vi "Periodic Tasks.vi"(8 "error in":errorcluster) -> ()   [LabVIEW 2016]
doc: "This VI runs in parallel to other tasks. It can contain as many user-defined periodic loops as you need. These can carry out PID or other sorts of timed response."
uses:
  <vilib>/Rock Robotics/WPI/Utilities/WPI_GetSetVariantRefNum.vi
  Robot Global Data.vi
  <vilib>/Rock Robotics/Network Tables/NT Write Numeric Array.vi
  <vilib>/Rock Robotics/Network Tables/NT Write Number.vi
  <vilib>/Rock Robotics/WPI/Solenoid/WPI_SolenoidValue.ctl
  <vilib>/Rock Robotics/WPI/Solenoid/WPI_SolenoidSetEnum.vi
panel:
  in  "z axis offset":dbl=0.10000000000000006
  out "Waveform Chart":dbl[][](graph)=[[-62.41187234999887, 0.0]]
  in  "Right False":dbl=0.3
  in  "Left False":dbl=0.7
  in  "Right True":dbl=0.7
  in  "Left-True":dbl=0.3 format="%#_13g"
  out "SensorPosRotations":dbl=1921.607142857143
  out "Motor output Plot 2":cluster{"Applied Throttle":dbl}(graph)
  out "Target RPM":dbl=5349.336450505878
  out "SensorRPM Velocity RPM 2":dbl
  in  "Ramp Rate 2":dbl
  in  "I Zone 2":dbl
  in  "D 2":dbl=-0.008
  in  "I 2":dbl=-0.027
  in  "P 2":dbl=20.0
  out "Applied Output 2":dbl
  out "Speed Closed Loop Plots":T1(graph)={"Sensor Velocity"=0.0, "Encoder Velocity"=0.0, "Encoder Position"=-53805.0}
  out "SensorPos (rotations)":dbl=-0.15048543689320387
  out "Motor output Plot":cluster{"Applied Throttle":dbl}(graph)
  out "Target Position (rotations)":dbl=-0.15274800672560607
  out "SensorRPM Velocity RPM":dbl
  in  "Ramp Rate":dbl=2.0
  in  "I Zone":dbl
  in  "F - Generally is zero for position-servo":dbl
  in  "D":dbl=0.45
  in  "I":dbl=0.0001
  in  "P":dbl=1.9
  out "Applied Output":dbl
  out "Position Closed Loop Plots":cluster{dbl, "Sensor Velocity":dbl}(graph)={1.352755905511811, "Sensor Velocity"=1.3564954682779455}
  out "rightDistance":dbl=27.365850000000002
  out "leftDistance":dbl=-30.4065
  # "Launcher Control"
  # "Turret Controls"
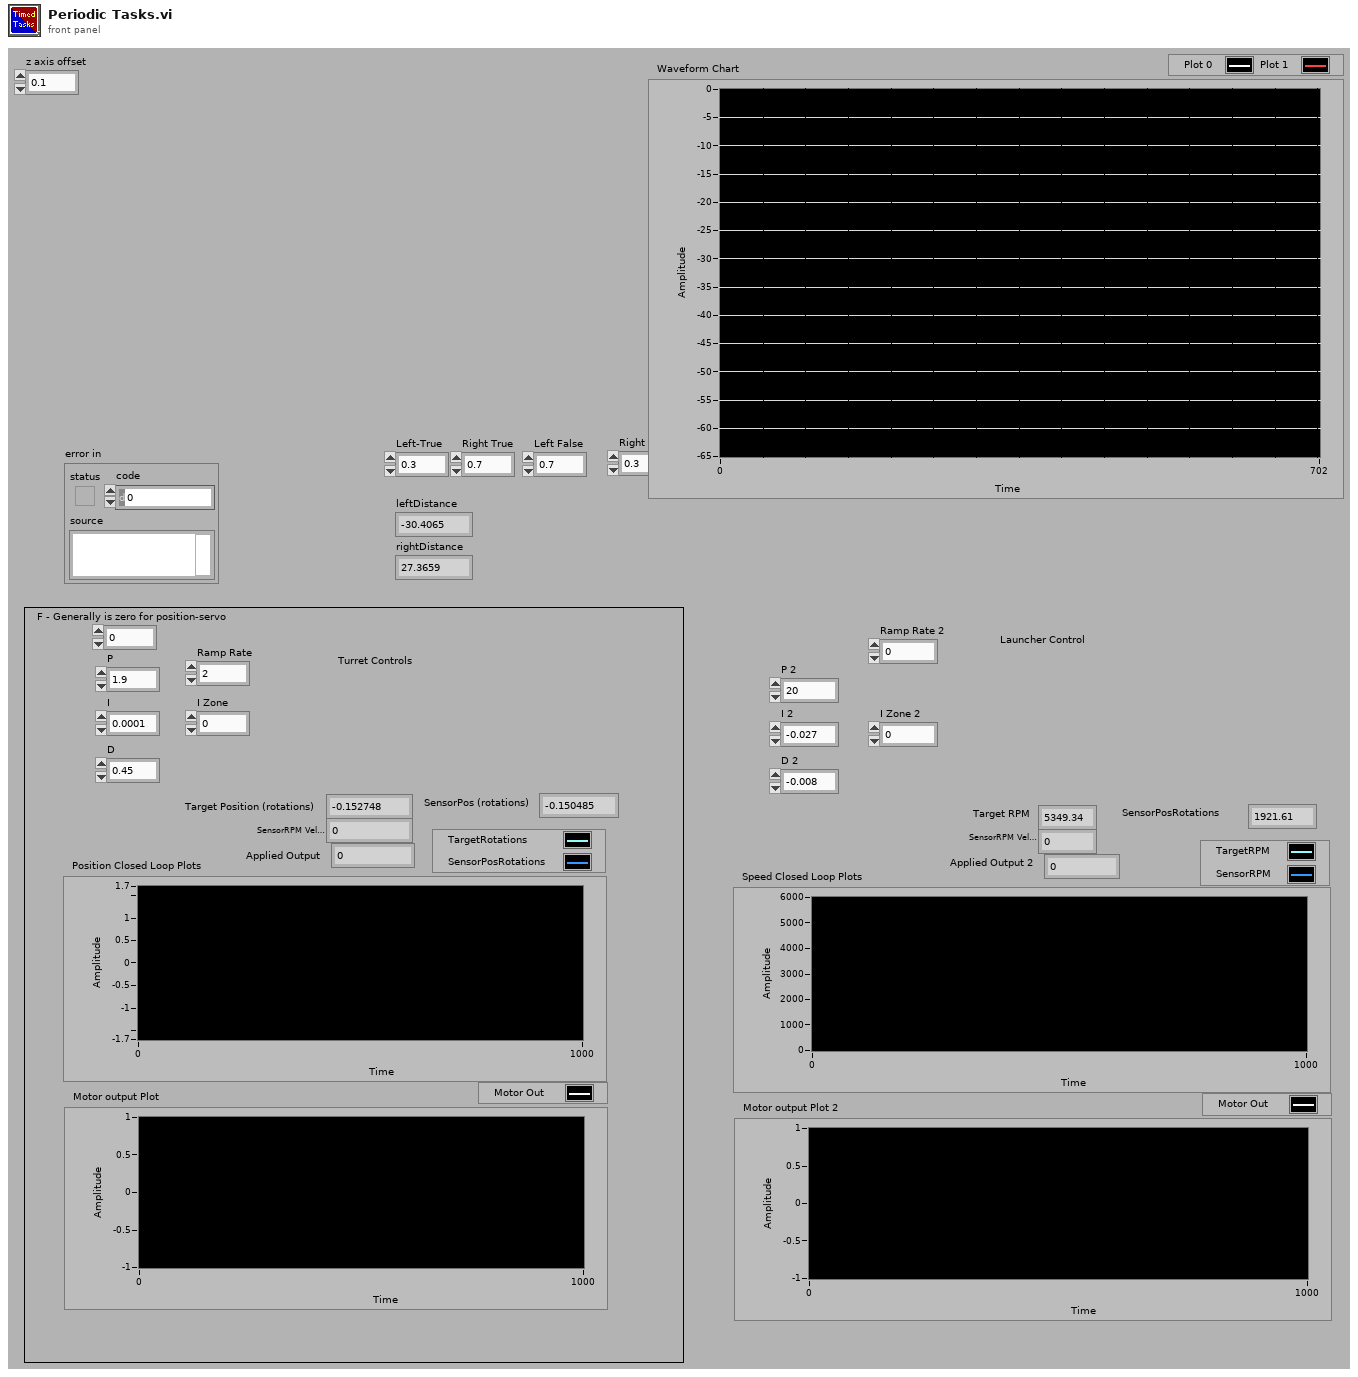
[diagram p1: front panel]
types:
  T1 = cluster{"Sensor Velocity":dbl, "Encoder Velocity":dbl, "Encoder Position":dbl}
  T2 = typedef "WPI_ServoDeviceRef.ctl" = cluster{"DeviceStatus":errorcluster, "PWM Channel":T3, "DeadBand":T4}
  T3 = typedef "FPGA_DIOPWMChannel.ctl" = enum8{"PWM 0", "PWM 1", "PWM 2", "PWM 3", "PWM 4", "PWM 5", "PWM 6", "PWM 7", "PWM 8", "PWM 9", "PWM MXP 0", "PWM MXP 1", "PWM MXP 2", "PWM MXP 3", "PWM MXP 4", "PWM MXP 5", "PWM MXP 6", "PWM MXP 7", "PWM MXP 8", "PWM MXP 9", "Invalid"}
  T4 = typedef "WPI_PWMDeadband.ctl" = cluster{"Name":string, "maxPositivePwm":i32, "minPositivePwm":i32, "centerPwm":i32, "maxNegativePwm":i32, "minNegativePwm":i32, "angularRange":u16}
  T5 = typedef "WPI_SolenoidValue.ctl" = enum16{"Off", "On", "Forward", "Reverse"}
  T6 = typedef "WPI_SolenoidDevRef.ctl" = cluster{"DevStatus":errorcluster, "Pneumatics Control Module":u8, "Forward Solenoid Channel":T7, "Reverse Solenoid Channel":T7}
  T7 = typedef "WPI_SolenoidChannel.ctl" = enum8{"Solenoid 0", "Solenoid 1", "Solenoid 2", "Solenoid 3", "Solenoid 4", "Solenoid 5", "Solenoid 6", "Solenoid 7", "Invalid"}
  T8 = typedef "WPI_MotorControlDeviceRef.ctl" = cluster{"DeviceStatus":errorcluster, "Type":T9, "PWM":cluster{"PWM Channel":T3, "DeadBand":T4}, "CAN":cluster{"Device Number":u8, "SetOutput VI Ref":variant, "GetOutput VI Ref":variant, "Enable VI Ref":variant, "Disable VI Ref":variant, "Data":variant}, "Invert":bool}
  T9 = typedef "WPI_MotorControlType.ctl" = enum16{"PWM", "CAN"}
  T10 = typedef "WPI_RobotDriveDevRef.ctl" = cluster{"DevStatus":errorcluster, "Motors[]":T8[], "Square Inputs":bool, "Max Output":dbl}
  T11 = typedef "WPI_GyroDevRef.ctl" = cluster{"DevStatus":errorcluster, "Analog Channel":T12, "Offset":dbl, "Gain (VoltsPerDegree/Second)":dbl, "Gyro Type":enum16{"Analog", "XRS450"}, "Handle":i32, "SPI Bus":T13, "Device Found":bool, "Sample Rate":dbl, "Calibrate On Open":bool}
  T12 = typedef "FPGA_AIChannel.ctl" = enum8{"AI 0", "AI 1", "AI 2", "AI 3", "AI MXP 0", "AI MXP 1", "AI MXP 2", "AI MXP 3", "Invalid"}
  T13 = typedef "spi_bus.ctl" = enum16{"SPI On-Board, CS0", "SPI On-Board, CS1", "SPI On-Board, CS2", "SPI On-Board, CS3", "SPI MXP", "Invalid"}
  T14 = typedef "WPI_EncoderDevRef.ctl" = cluster{"DevStatus":errorcluster, "EncoderIndex":T15, "CounterIndex":T16, "DistancePerCount":dbl, "Decoding Type":T17}
  T15 = typedef "FPGA_EncoderIdx.ctl" = enum8{"Enc 0", "Enc 1", "Enc 2", "Enc 3", "Enc 4", "Enc 5", "Enc 6", "Enc 7", "Invalid"}
  T16 = typedef "FPGA_CounterCtrSystemIndex.ctl" = enum8{"Ctr 0", "Ctr 1", "Ctr 2", "Ctr 3", "Ctr 4", "Ctr 5", "Ctr 6", "Ctr 7", "Invalid"}
  T17 = typedef "WPI_EncoderType.ctl" = enum16{"1x", "2x", "4x"}
  T18 = typedef "WPI_CANTalonSRX_GlobalStatus.ctl" = cluster{"Applied Throttle":dbl, "Module Enabled":bool, "CAN Error":errorcluster, "Closed Loop Error":dbl, "Forward Limit Switch Closed":bool, "Reverse Limit Switch Closed":bool, "Sensor Position":dbl, "Sensor Velocity":dbl, "Current":dbl, "Sticky Fault - Over Temp":bool, "Sticky Fault - Under Voltage":bool, "Sticky Fault - Forward Limit":bool, "Sticky Fault - Reverse Limit":bool, "Sticky Fault - Forward Soft Limit":bool, "Sticky Fault - Reverse Soft Limit":bool, "Brake is Enabled":bool, "Encoder Position":dbl, "Encoder Velocity":dbl, "Encoder Index Count":dbl, "Encoder A Pin State":bool, "Encoder B Pin State":bool, "Encoder Index Pin State":bool, "Analog In":dbl, "Analog In Velocity":dbl, "Temperature (C)":dbl, "Battery Voltage":dbl, "Control 5 Is Supported":bool, "Current Profile Slot Select":dbl, "Pos Div 8":bool, "Vel Div 4":bool, "Pulse Width Position":i32, "Pulse Width Velocity":i32, "Pulse Width Rise To Rise (us)":i32, "Pulse Width Rise To Fall (us)":i32, "Mot Prof Active Is Under Run":bool, "Mot Prof Active Has Under Run":bool, "Mot Prof Active Is Last":bool, "Mot Prof Active Velocity Only":bool, "Mot Prof Active Is Valid":bool, "Mot Prof Buffer Is Full":bool, "Mot Prof Active Profile Slot Select":i32, "Mot Prof NextID":i32, "Mot Prof Count":i32, "Mot Prof Active Velocity":dbl, "Mot Prof Active Position":dbl, "Mot Prof Output Enable":i32, "UsageFrame":u32, "Motion Magic Active Trajectory":cluster{"Velocity":dbl, "Position":dbl}}
  T19 = typedef "WPI_SwitchDevRef.ctl" = cluster{"DevStatus":errorcluster, "DIO Channel":T20, "CntIndex":T16, "Normally Closed":bool}
  T20 = typedef "FPGA_DIOChannel.ctl" = enum8{"DIO 0", "DIO 1", "DIO 2", "DIO 3", "DIO 4", "DIO 5", "DIO 6", "DIO 7", "DIO 8", "DIO 9", "DIO MXP 0", "DIO MXP 1", "DIO MXP 2", "DIO MXP 3", "DIO MXP 4", "DIO MXP 5", "DIO MXP 6", "DIO MXP 7", "DIO MXP 8", "DIO MXP 9", "DIO MXP 10", "DIO MXP 11", "DIO MXP 12", "DIO MXP 13", "DIO MXP 14", "DIO MXP 15", "SPI Port CS1", "SPI Port CS2", "SPI Port CS3", "SPI Port MISO", "SPI Port MOSI", "Invalid"}
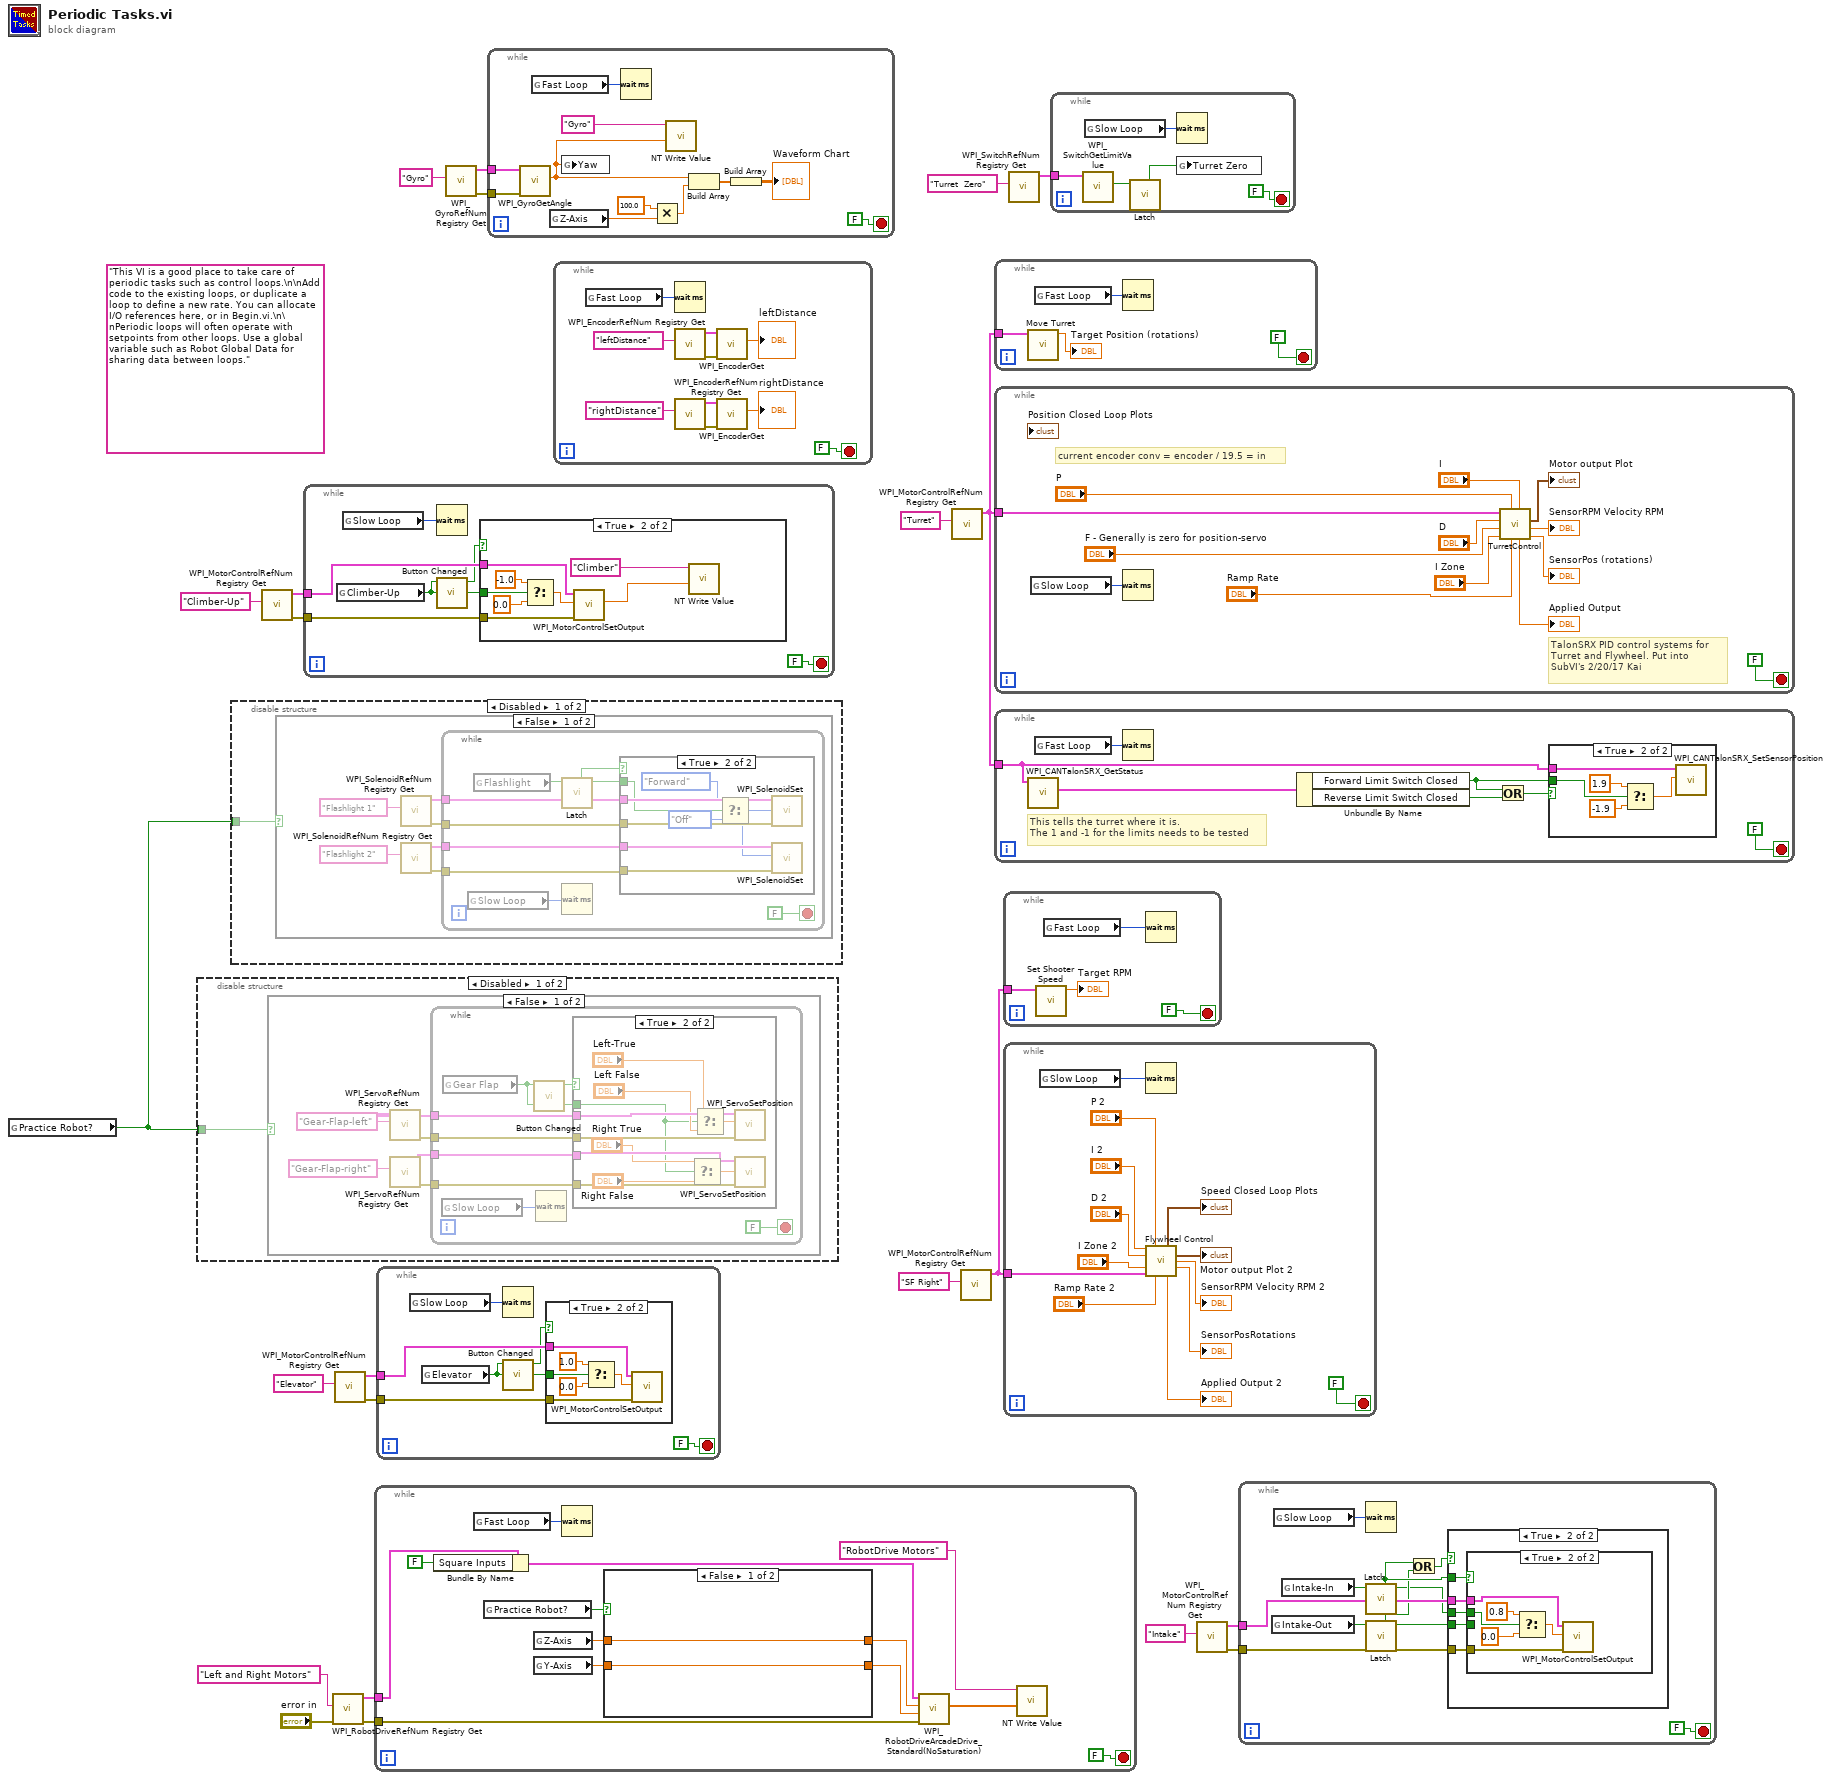
[diagram p0: block diagram]
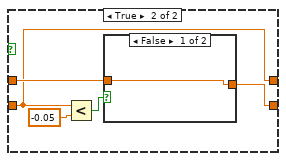
[diagram p10: hidden frame]
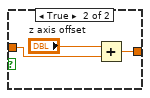
[diagram p11: hidden frame]
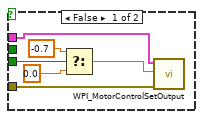
[diagram p14: hidden frame]
diagram:
  (unwired) "This VI is a good place to take care of periodic tasks such as control loops.\n\nAdd code to the existing loops, or duplicate a loop to define a new rate. You can allocate I/O references here, or in Begin.vi.\n\nPeriodic loops will often operate with setpoints from other loops. Use a global variable such as Robot Global Data for sharing data between loops."
  n1 = global read "Robot Global Data.vi" "Practice Robot?"() -> (w13:bool)
  n2 = disable-structure shown="Disabled" {
    disable-tunnel: w13 -> [w24 _]
    frame Disabled {
      n3 = case shown="False" w24 {
        frame False {
          n4 = call <vilib>:"WPI_ServoRefNum Registry Get.vi"("refnum name"="Gear-Flap-left") -> ("error out"=w27:errorcluster, "ServoDeviceRef"=w28:T2)  [unwired: 9 in]
          n5 = call <vilib>:"WPI_ServoRefNum Registry Get.vi"("refnum name"="Gear-Flap-right") -> ("error out"=w25:errorcluster, "ServoDeviceRef"=w26:T2)  [unwired: 9 in]
          n6 = while {
            tunnel: w28 -> [w38]
            tunnel: w27 -> [w37]
            tunnel: w26 -> [w36]
            tunnel: w25 -> [w35]
            stop <- FALSE stop-if-true
            n7 = global read "Robot Global Data.vi" "Slow Loop"() -> (w34:u32)
            n8 = global read "Robot Global Data.vi" "Gear Flap"() -> (w32:bool)
            n9 = call "Button Changed.vi"("In"=w32) -> ("button changed"=w33:bool)  [unwired: 10 in]
            n10 = Wait (ms)(milliseconds to wait=w34) -> ()  [unwired: 1 out]
            n11 = case shown="True" w33 {
              tunnel: w38 -> [_ w49]
              tunnel: w37 -> [_ w48]
              tunnel: w36 -> [_ w47]
              tunnel: w35 -> [_ w46]
              tunnel: w32 -> [_ w40]
              frame False {
              }
              frame True {
                n12 = Select(t="Right True", s=w40, f="Right False") -> (s? t:f=w45:dbl)
                n13 = Select(t="Left-True", s=w40, f="Left False") -> (s? t:f=w42:dbl)
                n14 = call <vilib>:"WPI_ServoSetPosition.vi"("error in (no error)"=w48, "Position"=w42, "ServoDeviceRef"=w49) -> ()  [unwired: 7 in, 2 out]
                n15 = call <vilib>:"WPI_ServoSetPosition.vi"("error in (no error)"=w46, "Position"=w45, "ServoDeviceRef"=w47) -> ()  [unwired: 7 in, 2 out]
              }
            }
          }
        }
        frame True {
        }
      }
    }
    frame Enabled {
    }
  }
  n16 = disable-structure shown="Disabled" {
    disable-tunnel: w13 -> [w50 _]
    frame Disabled {
      n17 = case shown="False" w50 {
        frame False {
          n18 = call <vilib>:"WPI_SolenoidRefNum Registry Get.vi"("refnum name"="Flashlight 1") -> ("error out"=w53:errorcluster, "SolenoidDevRef"=w54:T6)  [unwired: 9 in]
          n19 = call <vilib>:"WPI_SolenoidRefNum Registry Get.vi"("refnum name"="Flashlight 2") -> ("error out"=w51:errorcluster, "SolenoidDevRef"=w52:T6)  [unwired: 9 in]
          n20 = while {
            tunnel: w54 -> [w62]
            tunnel: w53 -> [w61]
            tunnel: w52 -> [w60]
            tunnel: w51 -> [w59]
            stop <- FALSE stop-if-true
            n21 = global read "Robot Global Data.vi" "Slow Loop"() -> (w58:u32)
            n22 = global read "Robot Global Data.vi" "Flashlight"() -> (w63:bool)
            n23 = call "Latch.vi"("In"=w63) -> ("Out"=w65:bool, "button pressed"=w64:bool)  [unwired: 9 in]
            n24 = Wait (ms)(milliseconds to wait=w58) -> ()  [unwired: 1 out]
            n25 = case shown="True" w64 {
              tunnel: w62 -> [_ w73]
              tunnel: w61 -> [_ w72]
              tunnel: w60 -> [_ w71]
              tunnel: w59 -> [_ w70]
              tunnel: w65 -> [_ w67]
              frame False {
              }
              frame True {
                n26 = Select(t=WPI_SolenoidValue."Forward" ("Value"), s=w67, f=WPI_SolenoidValue."Off" ("Value")) -> (s? t:f=w66:T5)
                n27 = call-poly <vilib>:"WPI_SolenoidSet.vi"("error in (no error)"=w72, "Value"=w66, "SolenoidDevRef"=w73) -> ()  [unwired: 7 in, 2 out]
                n28 = call-poly <vilib>:"WPI_SolenoidSet.vi"("error in (no error)"=w70, "Value"=w66, "SolenoidDevRef"=w71) -> ()  [unwired: 7 in, 2 out]
              }
            }
          }
        }
        frame True {
        }
      }
    }
    frame Enabled {
    }
  }
  n29 = call <vilib>:"WPI_MotorControlRefNum Registry Get.vi"("refnum name"="Climber-Up") -> ("error out"=w14:errorcluster, "MotorControlDevRef"=w15:T8)  [unwired: 9 in]
  n30 = while {
    tunnel: w15 -> [w79]
    tunnel: w14 -> [w78]
    stop <- FALSE stop-if-true
    n31 = global read "Robot Global Data.vi" "Climber-Up"() -> (w74:bool)
    n32 = global read "Robot Global Data.vi" "Slow Loop"() -> (w77:u32)
    n33 = Wait (ms)(milliseconds to wait=w77) -> ()  [unwired: 1 out]
    n34 = call "Button Changed.vi"("In"=w74) -> ("button changed"=w76:bool)  [unwired: 10 in]
    n35 = case shown="True" w76 {
      tunnel: w79 -> [_ w87]
      tunnel: w78 -> [_ w86]
      tunnel: w74 -> [_ w83]
      frame False {
      }
      frame True {
        n36 = Select(t=-1.0 ("Motor Output"), s=w83, f=0.0 ("Motor Output")) -> (s? t:f=w81:dbl)
        n37 = call <vilib>:"WPI_MotorControlSetOutput.vi"("error in (no error)"=w86, "Output"=w81, "MotorControlDevRef"=w87) -> ("Motor Output"=w80:dbl)  [unwired: 6 in, 2 out]
        n38 = call-poly <vilib>:"NT Write Value.vi"("Numeric"=w80, "Name"="Climber") -> ()  [unwired: 9 in, 1 out]
      }
    }
  }
  n39 = call <vilib>:"WPI_RobotDriveRefNum Registry Get.vi"("error in (no error)"="error in", "refnum name"="Left and Right Motors") -> ("error out"=w9:errorcluster, "RobotDriveDevRef"=w10:T10)  [unwired: 8 out]
  n40 = call <vilib>:"WPI_MotorControlRefNum Registry Get.vi"("refnum name"="Elevator") -> ("error out"=w12:errorcluster, "MotorControlDevRef"=w11:T8)  [unwired: 9 in]
  n41 = while {
    tunnel: w10 -> [w98]
    tunnel: w9 -> [w97]
    stop <- FALSE stop-if-true
    n42 = Bundle By Name(cluster=w98, "Square Inputs"=FALSE) -> (w94:T10)
    n43 = global read "Robot Global Data.vi" "Fast Loop"() -> (w95:u32)
    n44 = global read "Robot Global Data.vi" "Practice Robot?"() -> (w88:bool)
    n45 = global read "Robot Global Data.vi" "Z-Axis"() -> (w92:dbl)
    n46 = global read "Robot Global Data.vi" "Y-Axis"() -> (w90:dbl)
    n47 = Wait (ms)(milliseconds to wait=w95) -> ()  [unwired: 1 out]
    n48 = case shown="False" w88 {
      tunnel: w92 -> [w102 w107]
      tunnel: [w102 w105] -> w91
      tunnel: w90 -> [w101 w105]
      tunnel: [w101 w106] -> w89
      frame False {
      }
      frame True {
        n49 = Less?(x=w105, y=-0.05) -> (x < y?=w104:bool)
        n50 = case shown="False" w104 {
          tunnel: w107 -> [w108 w111]
          tunnel: [w108 w110] -> w106
          frame False {
          }
          frame True {
            n51 = Add(x="z axis offset", y=w111) -> (x+y=w110:dbl)
          }
        }
      }
    }
    n52 = call <vilib>:"WPI_RobotDriveArcadeDrive_Standard(NoSaturation).vi"("error in (no error)"=w97, "Y axis value"=w89, "X axis value"=w91, "RobotDriveDevRef"=w94) -> ("Motor Values"=w100:dbl[])  [unwired: 7 out]
    n53 = call-poly <vilib>:"NT Write Value.vi"("Numeric Array"=w100, "Name"="RobotDrive Motors") -> ()  [unwired: 9 in, 1 out]
  }
  n54 = while {
    tunnel: w12 -> [w117]
    tunnel: w11 -> [w116]
    stop <- FALSE stop-if-true
    n55 = global read "Robot Global Data.vi" "Slow Loop"() -> (w115:u32)
    n56 = global read "Robot Global Data.vi" "Elevator"() -> (w112:bool)
    n57 = Wait (ms)(milliseconds to wait=w115) -> ()  [unwired: 1 out]
    n58 = call "Button Changed.vi"("In"=w112) -> ("button changed"=w114:bool)  [unwired: 10 in]
    n59 = case shown="True" w114 {
      tunnel: w116 -> [_ w123]
      tunnel: w117 -> [_ w122]
      tunnel: w112 -> [_ w119]
      frame False {
      }
      frame True {
        n60 = Select(t=1.0 ("Output"), s=w119, f=0.0) -> (s? t:f=w121:dbl)
        n61 = call <vilib>:"WPI_MotorControlSetOutput.vi"("error in (no error)"=w122, "Output"=w121, "MotorControlDevRef"=w123) -> ()  [unwired: 6 in, 3 out]
      }
    }
  }
  n62 = call <vilib>:"WPI_GyroRefNum Registry Get.vi"("refnum name"="Gyro") -> ("error out"=w2:errorcluster, "GyroDevRef"=w3:T11)  [unwired: 9 in]
  n63 = while {
    tunnel: w3 -> [w127]
    tunnel: w2 -> [w126]
    stop <- FALSE stop-if-true
    n64 = call <vilib>:"WPI_GyroGetAngle.vi"("error in (no error)"=w126, "GyroDevRef"=w127) -> ("Angle"=w124:dbl)  [unwired: 6 in, 3 out]
    n65 = global read "Robot Global Data.vi" "Fast Loop"() -> (w133:u32)
    n66 = global read "Robot Global Data.vi" "Z-Axis"() -> (w132:dbl)
    n67 = global write "Robot Global Data.vi" "Yaw"(w124) -> ()
    n68 = Wait (ms)(milliseconds to wait=w133) -> ()  [unwired: 1 out]
    n69 = Multiply(x=100.0, y=w132) -> (x*y=w129:dbl)
    n70 = call-poly <vilib>:"NT Write Value.vi"("Numeric"=w124, "Name"="Gyro") -> ()  [unwired: 9 in, 1 out]
    n71 = Build Array(w124, w129) -> (w131:dbl[])
    n72 = Build Array(w131) -> (→"Waveform Chart":dbl[][])
  }
  n73 = while {
    stop <- FALSE stop-if-true
    n74 = global read "Robot Global Data.vi" "Fast Loop"() -> (w135:u32)
    n75 = Wait (ms)(milliseconds to wait=w135) -> ()  [unwired: 1 out]
    n76 = call <vilib>:"WPI_EncoderRefNum Registry Get.vi"("refnum name"="leftDistance") -> ("error out"=w144:errorcluster, "EncoderDevRef"=w143:T14)  [unwired: 9 in]
    n77 = call <vilib>:"WPI_EncoderRefNum Registry Get.vi"("refnum name"="rightDistance") -> ("error out"=w142:errorcluster, "EncoderDevRef"=w141:T14)  [unwired: 9 in]
    n78 = call <vilib>:"WPI_EncoderGet.vi"("error in (no error)"=w144, "EncoderDevRef"=w143) -> ("Distance"=→"leftDistance":dbl)  [unwired: 4 in, 5 out]
    n79 = call <vilib>:"WPI_EncoderGet.vi"("error in (no error)"=w142, "EncoderDevRef"=w141) -> ("Distance"=→"rightDistance":dbl)  [unwired: 4 in, 5 out]
  }
  n80 = call <vilib>:"WPI_MotorControlRefNum Registry Get.vi"("refnum name"="Turret") -> ("MotorControlDevRef"=w1:T8)  [unwired: 9 in, 1 out]
  n81 = call <vilib>:"WPI_MotorControlRefNum Registry Get.vi"("refnum name"="SF Right") -> ("MotorControlDevRef"=w5:T8)  [unwired: 9 in, 1 out]
  n82 = while {
    tunnel: w1 -> [w145]
    stop <- FALSE stop-if-true
    n83 = call "Move Turret.vi"("CAN Talon SRX Ref"=w145) -> ("Target X-value (norm)"=→"Target Position (rotations)":dbl)  [unwired: 10 in]
    n84 = global read "Robot Global Data.vi" "Fast Loop"() -> (w147:u32)
    n85 = Wait (ms)(milliseconds to wait=w147) -> ()  [unwired: 1 out]
  }
  n86 = while {
    tunnel: w1 -> [w149]
    stop <- FALSE stop-if-true
    # "current encoder conv = encoder / 19.5 = in"
    # "TalonSRX PID control systems for\nTurret and Flywheel. Put into \nSubVI's 2/20/17 Kai"
    n87 = global read "Robot Global Data.vi" "Slow Loop"() -> (w151:u32)
    n88 = Wait (ms)(milliseconds to wait=w151) -> ()  [unwired: 1 out]
    n89 = call "TurretControl.vi"("I"="I", "Ramp Rate"="Ramp Rate", "P"="P", "I Zone"="I Zone", "F - Generally is zero for position-servo"="F - Generally is zero for position-servo", "D"="D", "CAN Talon SRX Ref"=w149) -> ("SensorPos (rotations)"=→"SensorPos (rotations)":dbl, "SensorRPM Velocity RPM"=→"SensorRPM Velocity RPM":dbl, "Motor output Plot"=→"Motor output Plot":cluster{"Applied Throttle":dbl}, "Applied Output"=→"Applied Output":dbl)  [unwired: 1 in]
  }
  n90 = while {
    tunnel: w1 -> [w163]
    stop <- FALSE stop-if-true
    # "This tells the turret where it is.\nThe 1 and -1 for the limits needs to be tested"
    n91 = call <vilib>:"WPI_CANTalonSRX_GetStatus.vi"("CAN Talon SRX Ref"=w163) -> ("Talon SRX Status"=w166:T18)  [unwired: 8 in, 2 out]
    n92 = global read "Robot Global Data.vi" "Fast Loop"() -> (w168:u32)
    n93 = Wait (ms)(milliseconds to wait=w168) -> ()  [unwired: 1 out]
    n94 = Unbundle By Name(w166) -> ("Forward Limit Switch Closed"=w162:bool, "Reverse Limit Switch Closed"=w164:bool)
    n95 = Or(x=w162, y=w164) -> (x .or. y?=w165:bool)
    n96 = case shown="True" w165 {
      tunnel: w162 -> [_ w173]
      tunnel: w163 -> [_ w169]
      frame False {
      }
      frame True {
        n97 = Select(t=1.9, s=w173, f=-1.9) -> (s? t:f=w170:dbl)
        n98 = call <vilib>:"WPI_CANTalonSRX_SetSensorPosition.vi"("New Sensor Position"=w170, "CAN Talon SRX Ref"=w169) -> ()  [unwired: 8 in, 2 out]
      }
    }
  }
  n99 = while {
    tunnel: w5 -> [w174]
    stop <- FALSE stop-if-true
    n100 = call "Set Shooter Speed.vi"("CAN Talon SRX Ref"=w174) -> ("Flywheel RPM"=→"Target RPM":dbl)  [unwired: 10 in]
    n101 = global read "Robot Global Data.vi" "Fast Loop"() -> (w176:u32)
    n102 = Wait (ms)(milliseconds to wait=w176) -> ()  [unwired: 1 out]
  }
  n103 = while {
    tunnel: w5 -> [w179]
    stop <- FALSE stop-if-true
    n104 = global read "Robot Global Data.vi" "Slow Loop"() -> (w181:u32)
    n105 = Wait (ms)(milliseconds to wait=w181) -> ()  [unwired: 1 out]
    n106 = call "Flywheel Control.vi"("I in"="I 2", "P in"="P 2", "D in"="D 2", "I Zone in"="I Zone 2", "CAN Talon SRX Ref"=w179, "Ramp Rate in"="Ramp Rate 2") -> ("Speed Closed Loop Plots"=→"Speed Closed Loop Plots":T1, "Motor output Plot 2"=→"Motor output Plot 2":cluster{"Applied Throttle":dbl}, "SensorRPM Velocity RPM 2"=→"SensorRPM Velocity RPM 2":dbl, "SensorPosRotations"=→"SensorPosRotations":dbl, "Applied Output 2"=→"Applied Output 2":dbl)  [unwired: 5 in]
  }
  n107 = call <vilib>:"WPI_SwitchRefNum Registry Get.vi"("refnum name"="Turret  Zero") -> ("SwitchDevRef"=w8:T19)  [unwired: 9 in, 1 out]
  n108 = while {
    tunnel: w8 -> [w194]
    stop <- FALSE stop-if-true
    n109 = call <vilib>:"WPI_SwitchGetLimitValue.vi"("SwitchDevRef"=w194) -> ("Switch Pressed"=w195:bool)  [unwired: 8 in, 2 out]
    n110 = global read "Robot Global Data.vi" "Slow Loop"() -> (w192:u32)
    n111 = call "Latch.vi"("In"=w195) -> ("button pressed"=w191:bool)  [unwired: 9 in, 1 out]
    n112 = Wait (ms)(milliseconds to wait=w192) -> ()  [unwired: 1 out]
    n113 = global write "Robot Global Data.vi" "Turret Zero"(w191) -> ()
  }
  n114 = call <vilib>:"WPI_MotorControlRefNum Registry Get.vi"("refnum name"="Intake") -> ("error out"=w21:errorcluster, "MotorControlDevRef"=w22:T8)  [unwired: 9 in]
  n115 = while {
    tunnel: w22 -> [w204]
    tunnel: w21 -> [w203]
    stop <- FALSE stop-if-true
    n116 = global read "Robot Global Data.vi" "Intake-Out"() -> (w201:bool)
    n117 = global read "Robot Global Data.vi" "Slow Loop"() -> (w200:u32)
    n118 = global read "Robot Global Data.vi" "Intake-In"() -> (w202:bool)
    n119 = Wait (ms)(milliseconds to wait=w200) -> ()  [unwired: 1 out]
    n120 = call "Latch.vi"("In"=w202) -> ("Out"=w197:bool, "button pressed"=w199:bool)  [unwired: 9 in]
    n121 = call "Latch.vi"("In"=w201) -> ("Out"=w196:bool, "button pressed"=w198:bool)  [unwired: 9 in]
    n122 = Or(x=w199, y=w198) -> (x .or. y?=w205:bool)
    n123 = case shown="True" w205 {
      tunnel: w204 -> [_ w211]
      tunnel: w203 -> [_ w210]
      tunnel: w199 -> [_ w209]
      tunnel: w197 -> [_ w208]
      tunnel: w196 -> [_ w207]
      frame False {
      }
      frame True {
        n124 = case shown="True" w209 {
          tunnel: w211 -> [w216 w223]
          tunnel: w210 -> [w217 w222]
          tunnel: w208 -> [_ w219]
          tunnel: w207 -> [w212 _]
          frame False {
            n125 = Select(t=-0.7 ("Motor Output"), s=w212, f=0.0 ("Motor Output")) -> (s? t:f=w215:dbl)
            n126 = call <vilib>:"WPI_MotorControlSetOutput.vi"("error in (no error)"=w217, "Output"=w215, "MotorControlDevRef"=w216) -> ()  [unwired: 6 in, 3 out]
          }
          frame True {
            n127 = Select(t=0.8 ("Motor Output"), s=w219, f=0.0 ("Motor Output")) -> (s? t:f=w221:dbl)
            n128 = call <vilib>:"WPI_MotorControlSetOutput.vi"("error in (no error)"=w222, "Output"=w221, "MotorControlDevRef"=w223) -> ()  [unwired: 6 in, 3 out]
          }
        }
      }
    }
  }
